vi "indexed_cache_byte.vi"(3 "bool":bool, 4 "start_index":u8, 5 "index":u8) -> (1 "bool_byte":u8)   [LabVIEW 2018]
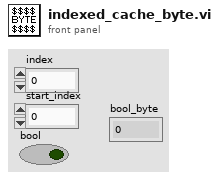
[diagram p1: front panel]
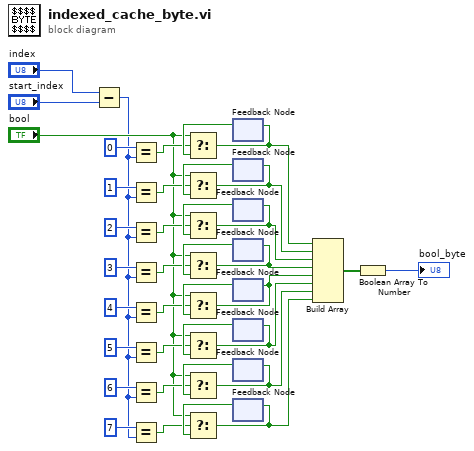
[diagram p0: block diagram]
diagram:
  n1 = Subtract(x="index", y="start_index") -> (x-y=w3:u8)
  n2 = Equal?(x=u8 0, y=w3) -> (x = y?=w37:bool)
  n3 = Equal?(x=u8 1, y=w3) -> (x = y?=w34:bool)
  n4 = Equal?(x=u8 2, y=w3) -> (x = y?=w31:bool)
  n5 = Equal?(x=u8 3, y=w3) -> (x = y?=w28:bool)
  n6 = Equal?(x=u8 4, y=w3) -> (x = y?=w25:bool)
  n7 = Equal?(x=u8 5, y=w3) -> (x = y?=w22:bool)
  n8 = Equal?(x=u8 6, y=w3) -> (x = y?=w19:bool)
  n9 = Equal?(x=u8 7, y=w3) -> (x = y?=w16:bool)
  n10 = feedback #1() -> (w38:bool)  [unwired: 1 in]
  n11 = Select(t="bool", s=w37, f=w38) -> (s? t:f=w9:bool)
  n12 = feedback-in #1(w9) -> ()
  n13 = feedback #2() -> (w35:bool)  [unwired: 1 in]
  n14 = Select(t="bool", s=w34, f=w35) -> (s? t:f=w10:bool)
  n15 = feedback-in #2(w10) -> ()
  n16 = feedback #3() -> (w32:bool)  [unwired: 1 in]
  n17 = Select(t="bool", s=w31, f=w32) -> (s? t:f=w12:bool)
  n18 = feedback-in #3(w12) -> ()
  n19 = feedback #4() -> (w29:bool)  [unwired: 1 in]
  n20 = Select(t="bool", s=w28, f=w29) -> (s? t:f=w14:bool)
  n21 = feedback-in #4(w14) -> ()
  n22 = feedback #5() -> (w26:bool)  [unwired: 1 in]
  n23 = Select(t="bool", s=w25, f=w26) -> (s? t:f=w13:bool)
  n24 = feedback-in #5(w13) -> ()
  n25 = feedback #6() -> (w23:bool)  [unwired: 1 in]
  n26 = Select(t="bool", s=w22, f=w23) -> (s? t:f=w11:bool)
  n27 = feedback-in #6(w11) -> ()
  n28 = feedback #7() -> (w20:bool)  [unwired: 1 in]
  n29 = Select(t="bool", s=w19, f=w20) -> (s? t:f=w8:bool)
  n30 = feedback-in #7(w8) -> ()
  n31 = feedback #8() -> (w17:bool)  [unwired: 1 in]
  n32 = Select(t="bool", s=w16, f=w17) -> (s? t:f=w7:bool)
  n33 = feedback-in #8(w7) -> ()
  n34 = Build Array(w9, w10, w12, w14, w13, w11, w8, w7) -> (w6:bool[])
  n35 = Boolean Array To Number(Boolean array=w6) -> (number=→"bool_byte":u8)
